vi "Teleop_Twist3ModeJohnny.vi"(8 "Angle":dbl, 9 "In drive deadband?":bool, 10 "Joy_R_Buttons":bool[](array[boolean]), 11 "Joy_R_Axes":dbl[](array[numeric])) -> (3 "Twist Output":dbl)   [LabVIEW 2017]
uses:
  TypeDefs/joyaxes.ctl
  TypeDefs/joybuttons.ctl
  <vilib>/ptbypt/NI_PtbyPt.lvlib
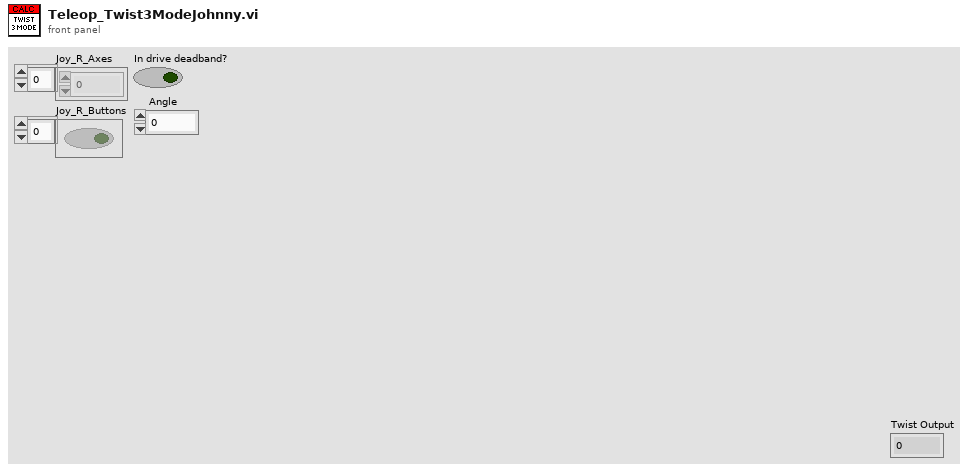
[diagram p1: front panel]
types:
  T1 = typedef "joyaxes.ctl" = enum16{"x axis", "y axis", "twist", "throttle"}
  T2 = typedef "joybuttons.ctl" = enum16{"Trigger", "Thumb", "Top3", "Top4", "Top5", "Top6", "Bottom7", "Bottom8", "Bottom9", "Bottom10", "Bottom11", "Bottom12", ""}
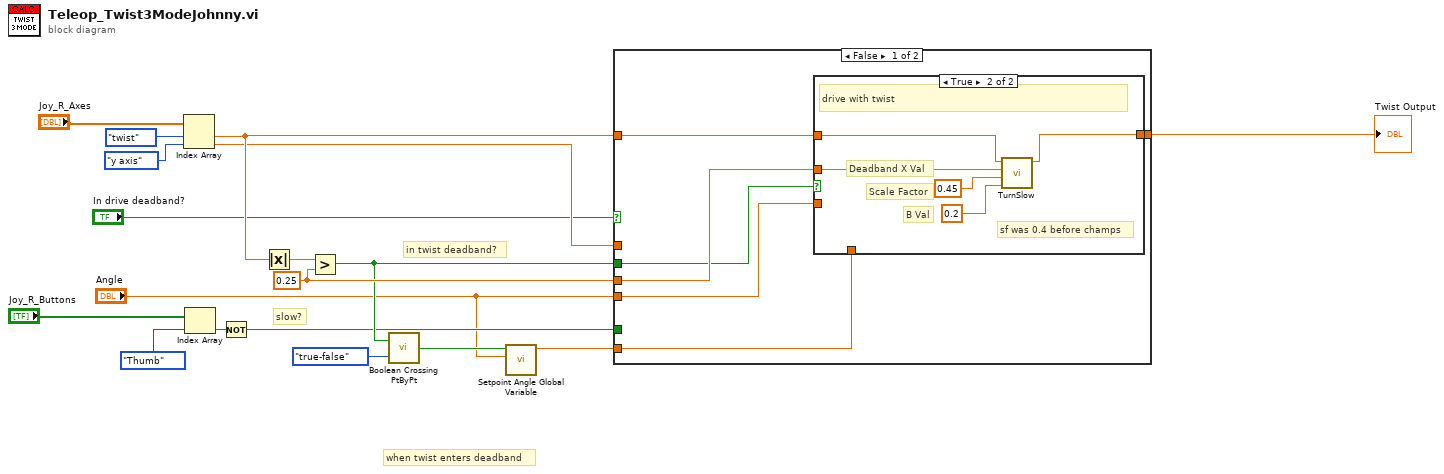
[diagram p0: block diagram]
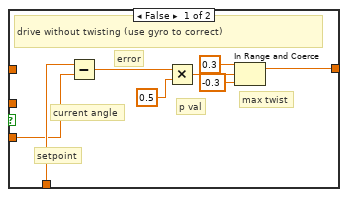
[diagram p2: hidden frame]
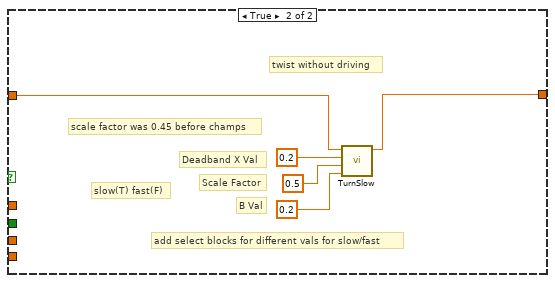
[diagram p3: hidden frame]
diagram:
  w15 = 0.25 ("y")
  # "in twist deadband?"
  # "slow?"
  # "when twist enters deadband"
  n1 = Index Array(array="Joy_R_Axes", index #1=joyaxes."twist" ("Enum"), index #2=joyaxes."y axis" ("Enum")) -> (element #1=w6:dbl, element #2=w5:dbl)
  n2 = Index Array(array="Joy_R_Buttons", index=joybuttons."Thumb" ("Enum")) -> (element=w10:bool)
  n3 = Not(x=w10) -> (.not. x?=w3:bool)
  n4 = Absolute Value(x=w6) -> (abs(x)=w17:dbl)
  n5 = Greater?(x=w17, y=w15) -> (0:w14:bool)
  n6 = call <vilib>:"Boolean Crossing PtByPt.vi"("direction"=enum16{"either", "false-true", "true-false"}."true-false", "input"=w14) -> ("crossing"=w13:bool)  [unwired: 1 in]
  n7 = call "Setpoint Angle Global Variable.vi"("Angle"="Angle", "T (Set) F (Get"=w13) -> ("Setpoint Angle"=w12:dbl)  [unwired: 9 in]
  n8 = case shown="False" "In drive deadband?" {
    tunnel: w6 -> [w23 w39]
    tunnel: w3 -> [_ _]
    tunnel: "Angle" -> [w20 _]
    tunnel: w5 -> [_ _]
    tunnel: [w24 w38] -> w18
    tunnel: w15 -> [w22 _]
    tunnel: w14 -> [w21 _]
    tunnel: w12 -> [w19 _]
    frame False {
      n9 = case shown="True" w21 {
        tunnel: [w25 w33] -> w24
        tunnel: w22 -> [_ w36]
        tunnel: w20 -> [w31 _]
        tunnel: w23 -> [_ w37]
        tunnel: w19 -> [w32 _]
        frame False {
          # "max twist"
          # "current angle"
          # "setpoint"
          # "error"
          # "p val"
          # "drive without twisting (use gyro to correct)"
          n10 = Subtract(x=w32, y=w31) -> (x-y=w30:dbl)
          n11 = Multiply(x=w30, y=0.5) -> (x*y=w28:dbl)
          n12 = In Range and Coerce(upper limit=0.3, x=w28, lower limit=-0.3) -> (coerced(x)=w25:dbl)  [unwired: 1 out]
        }
        frame True {
          # "sf was 0.4 before champs"
          # "drive with twist"
          # "B Val"
          # "Scale Factor"
          # "Deadband X Val"
          n13 = call "TurnSlow.vi"("b - value"=0.2, "Scale Factor"=0.45, "Deadband X value"=w36, "Input Twist"=w37) -> ("Twist Output"=w33:dbl)  [unwired: 7 in]
        }
      }
    }
    frame True {
      # "scale factor was 0.45 before champs"
      # "add select blocks for different vals for slow/fast"
      # "slow(T) fast(F)"
      # "B Val"
      # "Scale Factor"
      # "Deadband X Val"
      # "twist without driving"
      n14 = call "TurnSlow.vi"("b - value"=0.2 ("b value"), "Scale Factor"=0.5, "Deadband X value"=0.2, "Input Twist"=w39) -> ("Twist Output"=w38:dbl)  [unwired: 7 in]
    }
  }
  "Twist Output" <- w18
